vi "errorToStrings.vi"(8 "error in (no error)":errorcluster) -> (0 "error out":errorcluster, 2 "strings":string[](array[string]))   [LabVIEW 2013]
uses:
  <vilib>/Utility/error.llb/DialogType.ctl
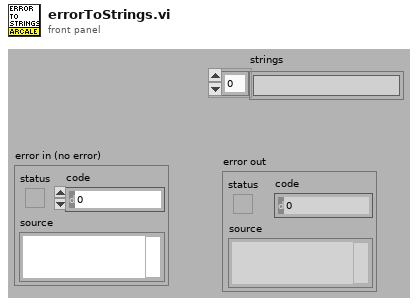
[diagram p1: front panel]
types:
  T1 = typedef "DialogType.ctl" = u16
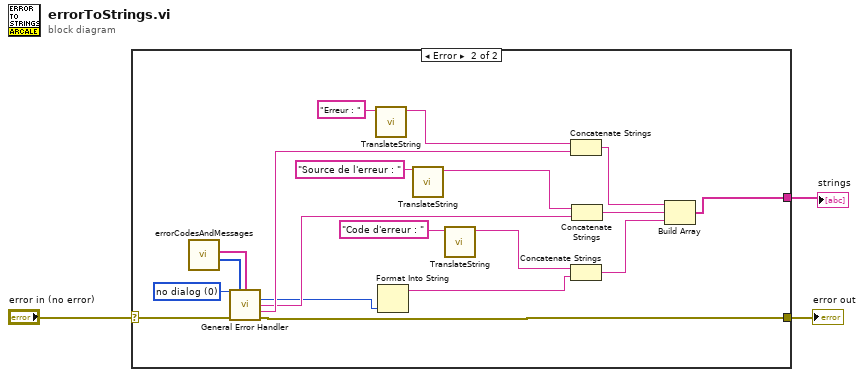
[diagram p0: block diagram]
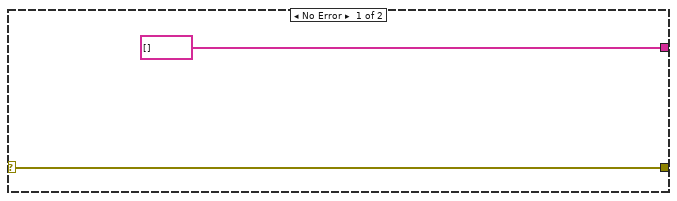
[diagram p2: hidden frame]
diagram:
  n1 = case shown="Error" "error in (no error)" {
    selector: "error in (no error)" -> [w5 w21]
    tunnel: [w5 w12] -> w2
    tunnel: [string[] [] ("strings") w13] -> w1
    frame No Error {
    }
    frame Error {
      w24 = T1 0 items=["no dialog", "OK message", "continue or stop message", "OK message + warnings", "continue/stop + warnings"] ("type of dialog (OK msg:1)")
      n2 = call "errorCodesAndMessages.vi"() -> ("errorCodes"=w23:i32[], "errorMessages"=w22:string[])  [unwired: 10 out]
      n3 = call <vilib>:"General Error Handler.vi"("[user-defined codes]"=w23, "[user-defined descriptions]"=w22, "type of dialog (OK msg:1)"=w24, "error in (no error)"=w21) -> ("code out"=w17:i32, "source out"=w19:string, "message"=w20:string, "error out"=w12:errorcluster)  [unwired: 8 out]
      n4 = call "TranslateString.vi"("String"="Erreur : " ("string")) -> ("Translated String"=w10:string)  [unwired: 9 in, 1 out]
      n5 = Format Into String(w17) -> (resulting string=w18:string)  [unwired: 3 in, 1 out]
      n6 = call "TranslateString.vi"("String"="Source de l'erreur : " ("string")) -> ("Translated String"=w8:string)  [unwired: 9 in, 1 out]
      n7 = call "TranslateString.vi"("String"="Code d'erreur : " ("string")) -> ("Translated String"=w6:string)  [unwired: 9 in, 1 out]
      n8 = Concatenate Strings(w10, w20) -> (w16:string)
      n9 = Concatenate Strings(w6, w18) -> (w14:string)
      n10 = Concatenate Strings(w8, w19) -> (w15:string)
      n11 = Build Array(w16, w15, w14) -> (w13:string[])
    }
  }
  "error out" <- w2
  "strings" <- w1
